vi "subLoadCommandlineArgs.vi"(9 "App.Args":string[](array[string])=["LabVIEW"], 11 "Options in":T1) -> (0 "error out":errorcluster, 1 "From command line?":bool, 2 "Pre-built libraries":refnum<class "ProjectItem.lvclass">[](array[class]), 3 "Options":T1, 4 "Active targets":string[](array[string]))   [LabVIEW 2019, in "SolutionBuilder.lvlib" / "SolutionBuilder.lvclass"]
uses:
  SolutionBuilder.lvclass
  Options.ctl
  ProjectItem/ProjectItem.lvclass
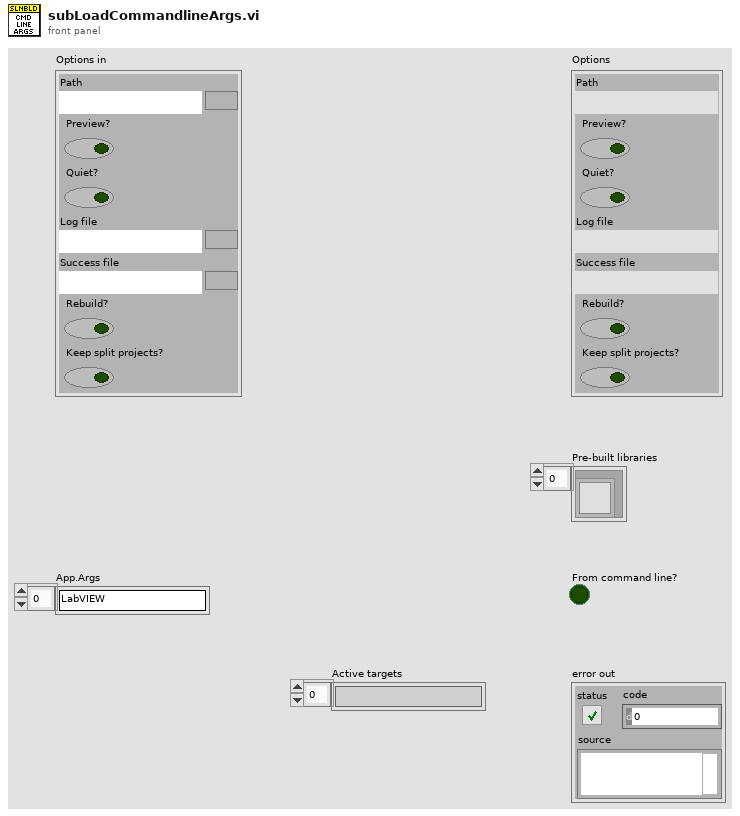
[diagram p1: front panel]
types:
  T1 = typedef "SolutionBuilder.lvlib/SolutionBuilder.lvclass/Options.ctl" = cluster{"Path":path, "Preview?":bool, "Quiet?":bool, "Log file":path, "Success file":path, "Rebuild?":bool, "Keep split projects?":bool}
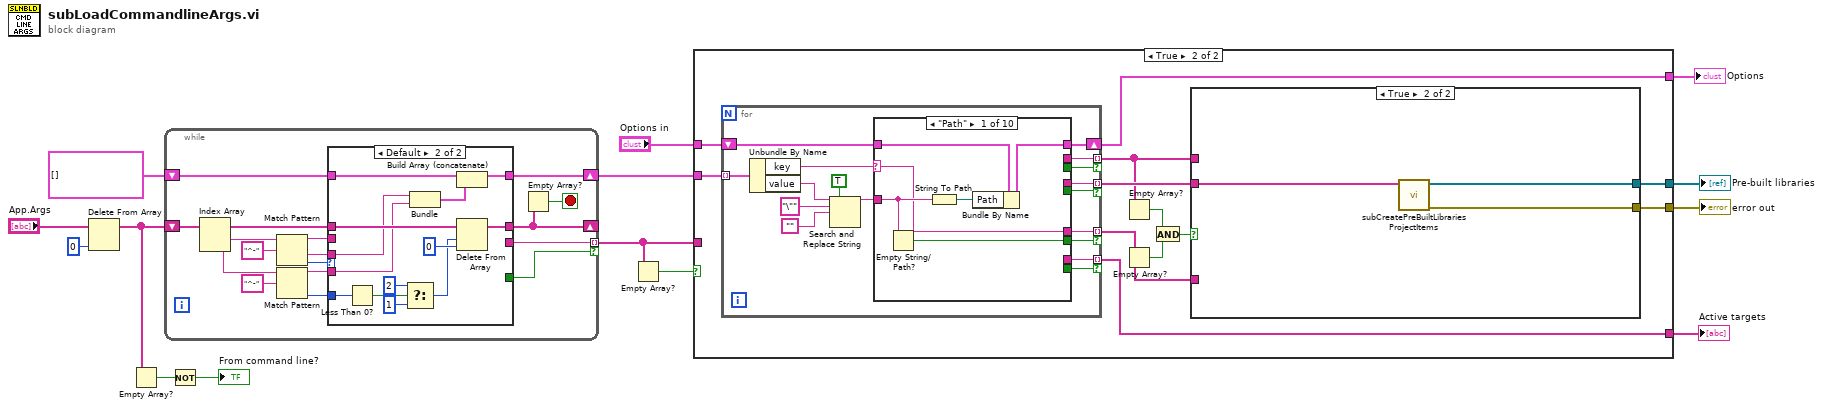
[diagram p0: block diagram]
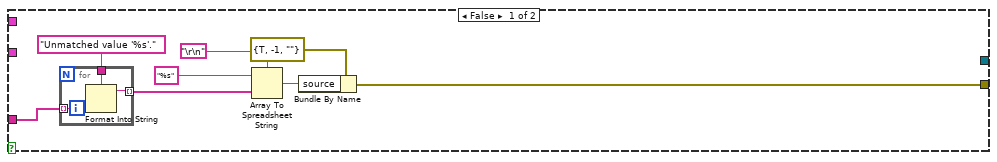
[diagram p2: hidden frame]
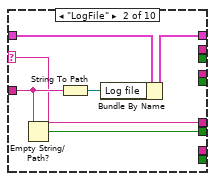
[diagram p3: hidden frame]
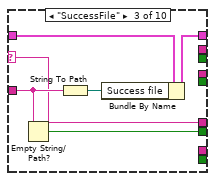
[diagram p4: hidden frame]
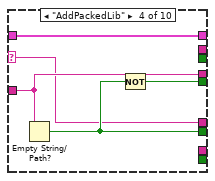
[diagram p5: hidden frame]
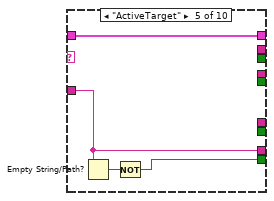
[diagram p6: hidden frame]
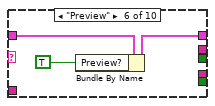
[diagram p7: hidden frame]
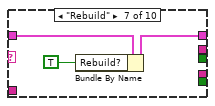
[diagram p8: hidden frame]
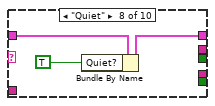
[diagram p9: hidden frame]
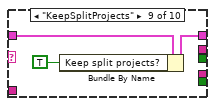
[diagram p10: hidden frame]
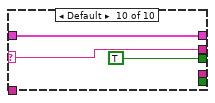
[diagram p11: hidden frame]
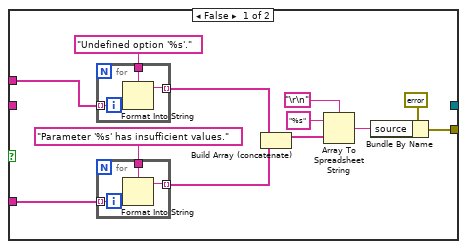
[diagram p12: hidden frame]
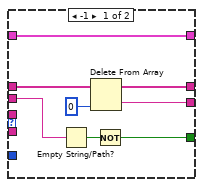
[diagram p13: hidden frame]
diagram:
  n1 = Delete From Array(array="App.Args", index=0) -> (array with subset deleted=w13:string[])  [unwired: 1 in, 1 out]
  n2 = Empty Array?(array=w13) -> (empty?=w12:bool)
  n3 = while {
    shift-right: [w19] -> _
    shift-left: w13 -> [w22]
    shift-right: [w20] -> w9
    shift-left: cluster{"key":string, "value":string}[] [] -> [w21]
    tunnel: [w17] -> w6 mode=indexing if=w16
    stop <- w18 stop-if-true
    n4 = Index Array(array=w22) -> (element #1=w30:string, element #2=w27:string)  [unwired: 2 in]
    n5 = Match Pattern(string=w30, regular expression="^-") -> (before substring=w15:string, after substring=w25:string, offset past match=w26:i32)  [unwired: 1 in, 1 out]
    n6 = Match Pattern(string=w27, regular expression="^-") -> (before substring=w24:string, offset past match=w23:i32)  [unwired: 1 in, 2 out]
    n7 = case shown="Default" w26 {
      tunnel: w25 -> [_ w43]
      tunnel: w24 -> [_ w42]
      tunnel: w23 -> [_ w51]
      tunnel: w22 -> [w37 w49]
      tunnel: [w36 w44] -> w19
      tunnel: w21 -> [w35 w41]
      tunnel: [w35 w39] -> w20
      tunnel: [w34 _] -> w17
      tunnel: [w31 _] -> w16
      tunnel: w15 -> [w33 _]
      frame -1 {
        n8 = Empty String/Path?(string/path=w33) -> (empty?=w32:bool)
        n9 = Delete From Array(array=w37, index=0) -> (deleted portion=w34:string, array with subset deleted=w36:string[])  [unwired: 1 in]
        n10 = Not(x=w32) -> (.not. x?=w31:bool)
      }
      frame Default {
        n11 = Less Than 0?(x=w51) -> (x < 0?=w50:bool)
        n12 = Select(t=2 ("length"), s=w50, f=1 ("length")) -> (s? t:f=w45:i32)
        n13 = Bundle(w43, w42) -> (w40:cluster{string, string})  [unwired: 1 in]
        n14 = Build Array (concatenate)(w41, w40) -> (w39:cluster{string, string}[])
        n15 = Delete From Array(array=w49, length=w45, index=0) -> (array with subset deleted=w44:string[])  [unwired: 1 out]
      }
    }
    n16 = Empty Array?(array=w19) -> (empty?=w18:bool)
  }
  n17 = Not(x=w12) -> (.not. x?=→"From command line?":bool)
  n18 = Empty Array?(array=w6) -> (empty?=w7:bool)
  n19 = case shown="True" w7 {
    tunnel: "Options in" -> [_ w74]
    tunnel: w9 -> [_ w73]
    tunnel: [w53 w70] -> w8
    tunnel: w6 -> [w54 _]
    tunnel: [_ w71] -> w5
    tunnel: [_ w69] -> w4
    tunnel: [_ w63] -> w2
    frame False {
      n20 = for {
        tunnel: w54 -> [w62] mode=indexing
        tunnel: [w61] -> w56 mode=indexing
        tunnel: "Unmatched value '%s'." ("format string") -> [w60]
        n21 = Format Into String(format string=w60, w62) -> (resulting string=w61:string)  [unwired: 2 in, 1 out]
      }
      n22 = Array To Spreadsheet String(delimiter (Tab)="\r\n", array=w56, 3:"%s" ("format string")) -> (spreadsheet string=w57:string)
      n23 = Bundle By Name(cluster=errorcluster {"status"=TRUE, "code"=-1, "source"=""} ("error out"), "source"=w57) -> (w53:errorcluster)
    }
    frame True {
      n24 = for {
        shift-right: [w90] -> w71
        shift-left: w74 -> [w91]
        tunnel: w73 -> [w89] mode=indexing
        tunnel: [w87] -> w72 mode=indexing if=w86
        tunnel: [w85] -> w64 mode=indexing if=w84
        tunnel: [w83] -> w68 mode=indexing if=w82
        tunnel: [w81] -> w63 mode=indexing if=w80
        n25 = Unbundle By Name(w89) -> ("key"=w88:string, "value"=w79:string)
        n26 = Search and Replace String(replace all?=TRUE ("replace all? (F)"), input string=w79, search string="\"", replace string="") -> (result string=w78:string)  [unwired: 4 in, 3 out]
        n27 = case shown="\"Path\"" w88 {
          selector: w88 -> [w93 w99 w105 w111 _ _ _ _ _ w132]
          tunnel: w91 -> [w97 w103 w109 w114 w118 w121 w124 w127 w130 w133]
          tunnel: w78 -> [w94 w100 w106 w113 w116 _ _ _ _ _]
          tunnel: [w96 w102 w108 w114 w118 w120 w123 w126 w129 w133] -> w90
          tunnel: [_ _ _ w113 _ _ _ _ _ _] -> w87
          tunnel: [_ _ _ w110 _ _ _ _ _ _] -> w86
          tunnel: [_ _ _ _ _ _ _ _ _ w132] -> w85
          tunnel: [_ _ _ _ _ _ _ _ _ TRUE] -> w84
          tunnel: [w93 w99 w105 w111 _ _ _ _ _ _] -> w83
          tunnel: [w92 w98 w104 w112 _ _ _ _ _ _] -> w82
          tunnel: [_ _ _ _ w116 _ _ _ _ _] -> w81
          tunnel: [_ _ _ _ w115 _ _ _ _ _] -> w80
          frame "Path" {
            n28 = Empty String/Path?(string/path=w94) -> (empty?=w92:bool)
            n29 = String To Path(string=w94) -> (path=w95:path)
            n30 = Bundle By Name(cluster=w97, "Path"=w95) -> (w96:T1)
          }
          frame "LogFile" {
            n31 = Empty String/Path?(string/path=w100) -> (empty?=w98:bool)
            n32 = String To Path(string=w100) -> (path=w101:path)
            n33 = Bundle By Name(cluster=w103, "Log file"=w101) -> (w102:T1)
          }
          frame "SuccessFile" {
            n34 = Empty String/Path?(string/path=w106) -> (empty?=w104:bool)
            n35 = String To Path(string=w106) -> (path=w107:path)
            n36 = Bundle By Name(cluster=w109, "Success file"=w107) -> (w108:T1)
          }
          frame "AddPackedLib" {
            n37 = Empty String/Path?(string/path=w113) -> (empty?=w112:bool)
            n38 = Not(x=w112) -> (.not. x?=w110:bool)
          }
          frame "ActiveTarget" {
            n39 = Empty String/Path?(string/path=w116) -> (empty?=w117:bool)
            n40 = Not(x=w117) -> (.not. x?=w115:bool)
          }
          frame "Preview" {
            n41 = Bundle By Name(cluster=w121, "Preview?"=TRUE) -> (w120:T1)
          }
          frame "Rebuild" {
            n42 = Bundle By Name(cluster=w124, "Rebuild?"=TRUE ("Preview?")) -> (w123:T1)
          }
          frame "Quiet" {
            n43 = Bundle By Name(cluster=w127, "Quiet?"=TRUE ("Preview?")) -> (w126:T1)
          }
          frame "KeepSplitProjects" {
            n44 = Bundle By Name(cluster=w130, "Keep split projects?"=TRUE ("Preview?")) -> (w129:T1)
          }
          frame Default {
          }
        }
      }
      n45 = Empty Array?(array=w64) -> (empty?=w66:bool)
      n46 = Empty Array?(array=w68) -> (empty?=w67:bool)
      n47 = And(x=w66, y=w67) -> (x .and. y?=w65:bool)
      n48 = case shown="True" w65 {
        tunnel: w72 -> [_ w154]
        tunnel: [w140 w152] -> w70
        tunnel: [_ w153] -> w69
        tunnel: w68 -> [w136 _]
        tunnel: w64 -> [w137 _]
        frame False {
          n49 = for {
            tunnel: w137 -> [w151] mode=indexing
            tunnel: [w150] -> w139 mode=indexing
            tunnel: "Undefined option '%s'." ("format string") -> [w149]
            n50 = Format Into String(format string=w149, w151) -> (resulting string=w150:string)  [unwired: 2 in, 1 out]
          }
          n51 = for {
            tunnel: w136 -> [w148] mode=indexing
            tunnel: [w147] -> w134 mode=indexing
            tunnel: "Parameter '%s' has insufficient values." ("format string") -> [w146]
            n52 = Format Into String(format string=w146, w148) -> (resulting string=w147:string)  [unwired: 2 in, 1 out]
          }
          n53 = Build Array (concatenate)(w139, w134) -> (w138:string[])
          n54 = Array To Spreadsheet String(delimiter (Tab)="\r\n", array=w138, 3:"%s" ("format string")) -> (spreadsheet string=w142:string)
          n55 = Bundle By Name(cluster=errorcluster {"status"=TRUE, "code"=-1, "source"=""} ("error out"), "source"=w142) -> (w140:errorcluster)
        }
        frame True {
          n56 = call "subCreatePreBuiltLibrariesProjectItems.vi"("Lib definition strings"=w154) -> ("error out"=w152:errorcluster, "Pre-built libraries"=w153:refnum<class "ProjectItem.lvclass">[])  [unwired: 9 in]
        }
      }
    }
  }
  "error out" <- w8
  "Options" <- w5
  "Pre-built libraries" <- w4
  "Active targets" <- w2
